vi "ECS - System - Engine Run Time.vi"(0 "Loop Period [ms]":u32) -> ()   [LabVIEW 2015, in "ECS-RT.lvlib"]
uses:
  ECS-RT.lvlib
  Typedefs/EPT/Engine Status.ctl
  Globals/RT Data.vi
  <vilib>/Utility/config.llb/Read Key (U32).vi
  <vilib>/Utility/config.llb/Write Key (U32).vi
  ECS-Shared.lvlib
  <vilib>/Utility/config.llb/NI_LVConfig.lvlib
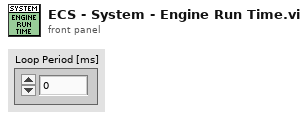
[diagram p1: front panel]
types:
  T1 = typedef "ECS-Shared.lvlib/Engine Status.ctl" = enum16{"OFF", "STALLED", "CRANKING", "RUNNING", "ACCEL", "DECEL", "SAFE"}
  T2 = typedef "NI_LVConfig.lvlib/Config Data RefNum.ctl" = refnum<k1>
  T3 = typedef "ECS-Shared.lvlib/RT Data.ctl" = cluster{"Refs":T4, "EPT":T6, "Raw Inputs":T8, "Control Inputs":T15, "Control Outputs":T17, "Raw Outputs":T20}
  T4 = typedef "ECS-Shared.lvlib/FPGA Refs.ctl" = cluster{"FPGA 1":T5, "FPGA 2":T5}
  T5 = typedef "ECS-Shared.lvlib/Generic FPGA Ref.ctl" = refnum<k20>
  T6 = typedef "ECS-Shared.lvlib/EPT Cluster.ctl" = cluster{"MaxCAD":sgl, "EPT Sim Enabled":bool, "EPTxData":T7}
  T7 = typedef "EPTx - RevA - RT.lvlib/EPTxData.ctl" = cluster{"Sync":bool, "CurrentCAD":sgl, "Speed [RPM]":sgl, "Config":bool, "Rcvg Primary":bool, "Stall":bool, "Overflow":bool, "Ratio Error":bool, "Pattern Error":bool, "Aux Warning":bool, "Watchdog Error":bool}
  T8 = typedef "ECS-Shared.lvlib/Raw Inputs.ctl" = cluster{"NI9752s":T9[], "NI9757s":T11[], "NI9411s":T12[], "NI9220s":T13[], "VRHalls":T14[]}
  T9 = typedef "ECS-Shared.lvlib/NI9752.ctl" = cluster{"Voltage [V]":sgl[], "Resistance [Ohm]":sgl[], "PPWData VR1":T10, "PPWData VR2":T10, "PPWData Hall1":T10, "PPWData Hall2":T10}
  T10 = typedef "ECS-Shared.lvlib/PPWData.ctl" = cluster{"Period":u32, "PulseWidth":u32, "Stopped":bool}
  T11 = typedef "ECS-Shared.lvlib/NI9757.ctl" = cluster{"UEGO1":cluster{"Lambda":sgl, "Phi":sgl, "AF_Ratio":sgl, "Ip":sgl, "Temp":sgl, "Hot":bool}, "UEGO2":cluster{"Lambda":sgl, "Phi":sgl, "AF_Ratio":sgl, "Ip":sgl, "Temp":sgl, "Hot":bool}, "EGO1":cluster{"Status":enum16{"COLD SENSOR", "FOULED SENSOR", "RICH", "LEAN"}, "SensorV":sgl}, "EGO2":cluster{"Status":enum16{"COLD SENSOR", "FOULED SENSOR", "RICH", "LEAN"}, "SensorV":sgl}, "EGO3":cluster{"Status":enum16{"COLD SENSOR", "FOULED SENSOR", "RICH", "LEAN"}, "SensorV":sgl}, "EGO4":cluster{"Status":enum16{"COLD SENSOR", "FOULED SENSOR", "RICH", "LEAN"}, "SensorV":sgl}}
  T12 = typedef "ECS-Shared.lvlib/NI9411.ctl" = cluster{"PPWData 0":T10, "PPWData 1":T10, "PPWData 2":T10, "PPWData 3":T10, "PPWData 4":T10, "PPWData 5":T10}
  T13 = typedef "ECS-Shared.lvlib/NI9220.ctl" = cluster{"AI 0":sgl, "AI 1":sgl, "AI 2":sgl, "AI 3":sgl, "AI 4":sgl, "AI 5":sgl, "AI 6":sgl, "AI 7":sgl, "AI 8":sgl, "AI 9":sgl, "AI 10":sgl, "AI 11":sgl, "AI 12":sgl, "AI 13":sgl, "AI 14":sgl, "AI 15":sgl}
  T14 = typedef "ECS-Shared.lvlib/VRHall.ctl" = cluster{"PPWData 0":T10, "PPWData 1":T10, "PPWData 2":T10, "PPWData 3":T10, "PPWData 4":T10, "PPWData 5":T10}
  T15 = typedef "ECS-Shared.lvlib/Control Inputs.ctl" = cluster{"Engine Speed [RPM]":sgl, "Engine Status":T1, "Load Control \nMode":T16, "dt(s)":sgl, "Number of Cylinders":u8, "Engine Displacement [cc]":sgl, "StoichAFR":sgl, "Q.LHV Fuel [kJ/kg]":sgl, "BattV PSU [V]":sgl, "12V PSU [V]":sgl, "5V PSU [V]":sgl, "Pedal Position [%]":sgl, "Oil Pressure [kPa]":sgl, "Oil Temp [C]":sgl, "Oil Level [%]":sgl, "Engine Coolant Temp (ECT) [C]":sgl, "Engine Coolant Pressure [kPa]":sgl, "Rail Pressure [bar]":sgl, "Fuel Pressure [kPa]":sgl, "Fuel Temp [C]":sgl, "Vacuum Pressure [kPa]":sgl, "Throttle Position [%]":sgl, "Cam1 Advance [CAD]":sgl, "Cam2 Advance [CAD]":sgl, "Cam3 Advance [CAD]":sgl, "Cam4 Advance [CAD]":sgl, "CA50 Control Output [CAD]":sgl[], "CA50 Control Output Valid":bool[], "Intake Air Temp (IAT) [C]":sgl, "Barometric Air Pressure [kPa]":sgl, "Intake Air Rel. Humidity [%]":sgl, "Mass Air Flow (MAF) [kg/hr]":sgl, "Turbo Inlet Air Pressure [kPa]":sgl, "Turbo Inlet Air Temp [C]":sgl, "Turbo Outlet Air Pressure [kPa]":sgl, "Turbo Outlet Air Temp [C]":sgl, "CAC Outlet Pressure [kPa]":sgl, "CAC Outlet Temp [C]":sgl, "Intake Manifold Pressure (MAP) [kPa]":sgl, "Intake Manifold Temp (MAT) [C]":sgl, "Exhaust Manifold Pressure [kPa]":sgl, "Exhaust Manifold Temp [C]":sgl, "HighP EGR Cooler Outlet Pressure [kPa]":sgl, "HighP EGR Cooler Outlet Temp [C]":sgl, "HighP EGR Differential Pressure [kPa]":sgl, "HighP EGR Valve Position [%]":sgl, "Turbo Outlet Exhaust Pressure [kPa]":sgl, "Turbo Outlet Exhaust Temp [C]":sgl, "VGT Position 1 [%]":sgl, "VGT Position 2 [%]":sgl, "Turbo Speed 1 [RPM]":sgl, "Turbo Speed 2 [RPM]":sgl, "LowP EGR Differential Pressure [kPa]":sgl, "LowP EGR Valve Position [%]":sgl, "UEGO1Lambda":sgl, "UEGO1_Hot":bool, "UEGO2Lambda":sgl, "UEGO2_Hot":bool, "Knock Intensity":sgl[], "Knock":bool[]}
  T16 = typedef "ECS-Shared.lvlib/Load Control Mode.ctl" = enum16{"No Governor", "Min Speed Governor", "Max Speed Governor"}
  T17 = typedef "ECS-Shared.lvlib/Control Outputs.ctl" = cluster{"Pedal Desired [%]":sgl, "MEP Desired [bar]":sgl, "Fuel Desired [mg/cyc]":sgl, "Intake MAP Desired [kPa]":sgl, "Cam1 Advance Setpoint [CAD]":sgl, "Cam2 Advance Setpoint [CAD]":sgl, "HighP EGR Position Setpoint [%Open]":sgl, "LowP EGR Position Setpoint [%Open]":sgl, "Rail Pressure Setpoint [bar]":sgl, "Wastegate1 Position Setpoint [%Open]":sgl, "Wastegate2 Position Setpoint [%Open]":sgl, "VGT1 Position Setpoint [%Open]":sgl, "VGT2 Position Setpoint [%Open]":sgl, "Throttle1 Position Setpoint [%Open]":sgl, "Throttle2 Position Setpoint [%Open]":sgl, "TurboBPV Position Setpoint [%Open]":sgl, "Spark Dwells [msec]":sgl[], "Spark Timings [DBTDC]":sgl[], "PFI Quantities [mg/inj]":sgl[], "PFI Timings [DBTDC]":sgl[], "DI Quantities [mg/inj]":T18[], "DI Timings [DBTDC]":T19[]}
  T18 = typedef "ECS-Shared.lvlib/Injection Quantity.ctl" = cluster{"Pilot1Quantity [mg/inj]":sgl, "Pilot2Quantity [mg/inj]":sgl, "MainQuantity [mg/inj]":sgl, "Post1Quantity [mg/inj]":sgl, "Post2Quantity [mg/inj]":sgl}
  T19 = typedef "ECS-Shared.lvlib/Injection Timing.ctl" = cluster{"Pilot1SOI [DBTDC]":sgl, "Pilot2SOI [DBTDC]":sgl, "MainSOI [DBTDC]":sgl, "Post1SOI [DBTDC]":sgl, "Post2SOI [DBTDC]":sgl}
  T20 = typedef "ECS-Shared.lvlib/Raw Outputs.ctl" = cluster{"9751-1":T21, "9751-2":T21, "9751-3":T21, "9751-4":T21, "9754-1":T23, "9754-2":T23, "9758-1":T25, "9758-2":T25, "9759-1":T28}
  T21 = typedef "ECS-Shared.lvlib/NI9751.ctl" = cluster{"DI1":T22, "DI2":T22, "DI3":T22}
  T22 = typedef "ECS-Shared.lvlib/DI.ctl" = cluster{"Window_Start (DBTDC)":sgl, "Window_End (DBTDC)":sgl, "Enable_Inj1":bool, "Duration_Inj1 (msec)":sgl, "Timing_Inj1 (DBTDC)":sgl, "Enable_Inj2":bool, "Duration_Inj2 (msec)":sgl, "Timing_Inj2 (DBTDC)":sgl, "Enable_Inj3":bool, "Duration_Inj3 (msec)":sgl, "Timing_Inj3 (DBTDC)":sgl, "Enable_Inj4":bool, "Duration_Inj4 (msec)":sgl, "Timing_Inj4 (DBTDC)":sgl, "Enable_Inj5":bool, "Duration_Inj5 (msec)":sgl, "Timing_Inj5 (DBTDC)":sgl}
  T23 = typedef "ECS-Shared.lvlib/NI9754.ctl" = cluster{"ESTTL 1":T24, "ESTTL 2":T24, "ESTTL 3":T24, "ESTTL 4":T24, "ESTTL 5":T24, "ESTTL 6":T24, "ESTTL 7":T24, "ESTTL 8":T24}
  T24 = typedef "ECS-Shared.lvlib/ESTTL.ctl" = cluster{"Timing (DBTDC)":sgl, "Dwell (ms)":sgl}
  T25 = typedef "ECS-Shared.lvlib/NI9758.ctl" = cluster{"LS 1":T26, "LS 2":T26, "LS 3":T26, "LS 4":T26, "PFI 1":T27, "PFI 2":T27, "PFI 3":T27, "PFI 4":T27}
  T26 = typedef "ECS-Shared.lvlib/LS.ctl" = cluster{"Enable":bool, "Freq [Hz]":sgl, "DutyCyc [%]":sgl}
  T27 = typedef "ECS-Shared.lvlib/PFI.ctl" = cluster{"Position Mode":bool, "Timing (DBTDC)":sgl, "Pulse Width (ms)":sgl}
  T28 = typedef "ECS-Shared.lvlib/NI9759.ctl" = cluster{"THR1-1 DC [%]":sgl, "THR1-1 Setpoint [% Open]":sgl, "THR1-2 DC [%]":sgl, "THR1-2 Setpoint [% Open]":sgl}
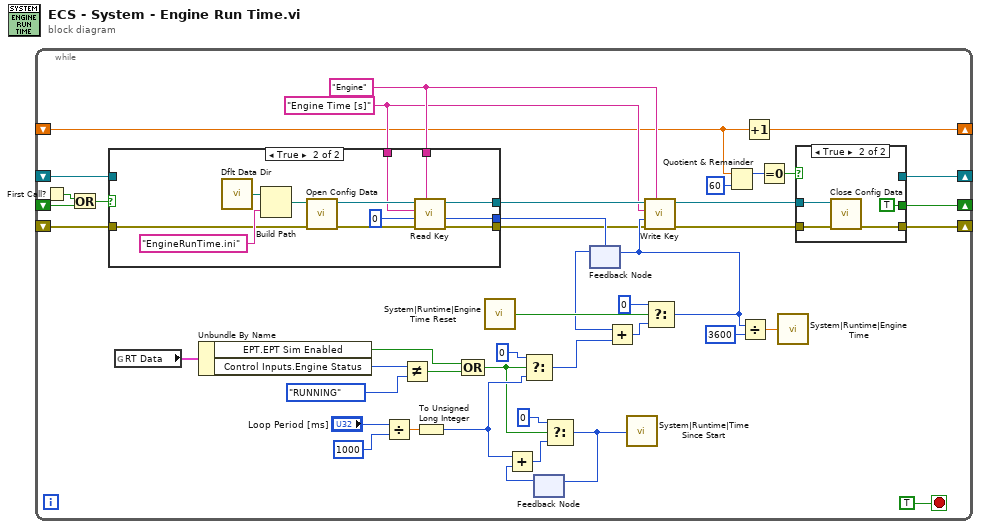
[diagram p0: block diagram]
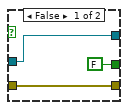
[diagram p2: hidden frame]
diagram:
  n1 = while {
    shift-right: [w25] -> _
    shift-left: _ -> [w13]
    shift-right: [w15] -> _
    shift-left: _ -> [w12]
    shift-right: [w11] -> _
    shift-left: _ -> [w10]
    shift-right: [w8] -> _
    shift-left: _ -> [w9]
    stop <- TRUE stop-if-true
    w19 = "Engine Time [s]" ("key")
    w20 = "Engine" ("section")
    n2 = First Call?() -> (First Call?: T/F=w14:bool)
    n3 = Or(x=w14, y=w13) -> (x .or. y?=w24:bool)
    n4 = case shown="True" w24 {
      tunnel: [_ w64] -> w29
      tunnel: [w52 w62] -> w22
      tunnel: w19 -> [_ w61]
      tunnel: w20 -> [_ w60]
      tunnel: [w53 w55] -> w17
      tunnel: w12 -> [w53 w54]
      tunnel: w10 -> [w52 _]
      frame False {
      }
      frame True {
        n5 = call <vilib>:"Dflt Data Dir.vi"() -> ("App:Default Data Directory"=w59:path)
        n6 = Build Path(base path=w59, name or relative path="EngineRunTime.ini" ("section")) -> (appended path=w57:path)
        n7 = call <vilib>:"Open Config Data.vi"("error in (no error)"=w54, "configuration file path"=w57) -> ("error out"=w56:errorcluster, "refnum"=w65:T2)  [unwired: 7 in, 1 out]
        n8 = call-poly <vilib>:"Read Key.vi"("section"=w60, "error in (no error)"=w56, "default value"=u32 0, "key"=w61, "refnum"=w65) -> ("error out"=w55:errorcluster, "value"=w64:u32, "refnum out"=w62:T2)  [unwired: 3 in, 1 out]
      }
    }
    n9 = global read "RT Data.vi" "RT Data"() -> (w4:T3)
    n10 = Unbundle By Name(w4) -> ("EPT.EPT Sim Enabled"=w6:bool, "Control Inputs.Engine Status"=w5:T1)
    n11 = Divide(x="Loop Period [ms]", y=u32 1000) -> (x/y=w38:dbl)
    n12 = Not Equal?(x=w5, y=Engine_Status."RUNNING") -> (x != y?=w3:bool)
    n13 = To Unsigned Long Integer(number=w38) -> (unsigned 32bit integer=w31:u32)
    n14 = Compound Arithmetic op=OR(w6, w3) -> (w1:bool)
    n15 = call "System|Runtime|Engine Time Reset"() -> ("Value"=w43:bool)
    n16 = Select(t=u32 0, s=w1, f=w31) -> (s? t:f=w40:u32)
    n17 = feedback #1() -> (w34:u32)  [unwired: 1 in]
    n18 = Add(x=w31, y=w34) -> (x+y=w33:u32)
    n19 = Select(t=u32 0, s=w1, f=w33) -> (s? t:f=w35:u32)
    n20 = feedback-in #1(w35) -> ()
    n21 = feedback #2(w29) -> (w30:u32)
    n22 = Add(x=w30, y=w40) -> (x+y=w42:u32)
    n23 = call "System|Runtime|Time Since Start"("Value"=w35) -> ()
    n24 = Select(t=u32 0, s=w43, f=w42) -> (s? t:f=w18:u32)
    n25 = feedback-in #2(w18) -> ()
    n26 = call-poly <vilib>:"Write Key.vi"("section"=w20, "error in (no error)"=w17, "value"=w18, "key"=w19, "refnum"=w22) -> ("error out"=w16:errorcluster, "refnum out"=w21:T2)  [unwired: 4 in, 1 out]
    n27 = Quotient & Remainder(x=w9, y=u64 60) -> (x-y*floor(x/y)=w27:u64)  [unwired: 1 out]
    n28 = Divide(x=w18, y=u32 3600) -> (x/y=w36:dbl)
    n29 = Increment(x=w9) -> (x+1=w8:dbl)
    n30 = Equal To 0?(x=w27) -> (x = 0?=w26:bool)
    n31 = call "System|Runtime|Engine Time"("Value"=w36) -> ()
    n32 = case shown="True" w26 {
      tunnel: w21 -> [w45 w50]
      tunnel: [FALSE TRUE] -> w25
      tunnel: w16 -> [w46 w49]
      tunnel: [w46 w48] -> w15
      tunnel: [w45 _] -> w11
      frame False {
      }
      frame True {
        n33 = call <vilib>:"Close Config Data.vi"("error in (no error)"=w49, "refnum"=w50) -> ("error out"=w48:errorcluster)  [unwired: 8 in, 1 out]
      }
    }
  }
